vi "Joint_Test.vi"(0 "Left_Joystick_Y":dbl, 1 "RT_Pressed":bool) -> ()   [LabVIEW 2018]
uses:
  Subsytems/Intake_Joint/Intake_Joint_Notifier.ctl
  Subsytems/Intake_Joint/Intake_Joint_Control_Type.ctl
  Global_Variables/Intake_Joint_Globals.vi
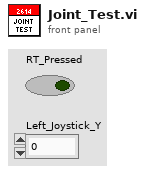
[diagram p1: front panel]
types:
  T1 = typedef "Intake_Joint_Notifier.ctl" = cluster{"Intake_Joint_Control_Type":T2, "Manual_Joint_Up":bool, "Manual_Joint_Down":bool}
  T2 = typedef "Intake_Joint_Control_Type.ctl" = enum16{"No_Op", "Manual_Joint_Up", "Manual_Joint_Down", "Manual_Position_Control"}
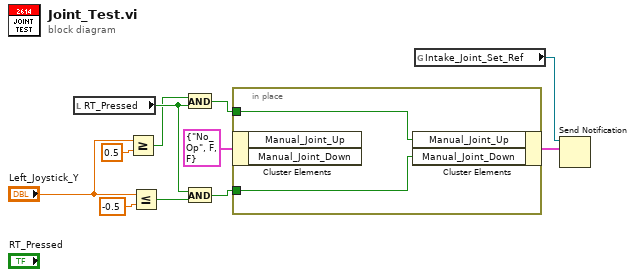
[diagram p0: block diagram]
diagram:
  n1 = local read "RT_Pressed"() -> (w5:bool)
  n2 = Greater Or Equal?(x="Left_Joystick_Y", y=0.5) -> (x >= y?=w3:bool)
  n3 = Less Or Equal?(x="Left_Joystick_Y", y=-0.5) -> (x <= y?=w4:bool)
  n4 = And(x=w3, y=w5) -> (x .and. y?=w2:bool)
  n5 = And(x=w5, y=w4) -> (x .and. y?=w1:bool)
  n6 = in-place {
    in-place-border: w2 -> [w13]
    in-place-border: w1 -> [w12]
    n7 = in-place-cluster #1(T1 {"Intake_Joint_Control_Type"=enum."No_Op", "Manual_Joint_Up"=FALSE, "Manual_Joint_Down"=FALSE} ("Intake_Joint_Notifier")) -> ()  [unwired: 2 out]
    n8 = in-place-cluster #1("Manual_Joint_Up"=w13, "Manual_Joint_Down"=w12) -> (w11:T1)
  }
  n9 = global read "Intake_Joint_Globals.vi" "Intake_Joint_Set_Ref"() -> (w9:refnum<notifier>)
  n10 = Send Notification(notification=w11, notifier=w9) -> ()  [unwired: 1 in, 2 out]
